vi "Format Name.vi"(11 "Sheet Name":string) -> (3 "Formatted Sheet Name":string)   [LabVIEW 2019, in "Open Xml.lvlib"]
uses:
  Open Xml.lvlib
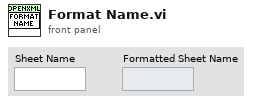
[diagram p1: front panel]
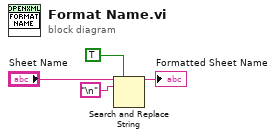
[diagram p0: block diagram]
diagram:
  n1 = Search and Replace String(replace all?=TRUE ("replace all? (F)"), input string="Sheet Name", search string="\n") -> (result string=→"Formatted Sheet Name":string)  [unwired: 5 in, 3 out]
